vi "Generate Simulated Data v2.0.vi"(0 "Sample_Rate":dbl, 1 "A_1X":dbl, 5 "Total_Samples in":i64, 7 "Samples":i32, 9 "f_1X":dbl, 11 "error in (no error)":errorcluster, 12 "A_2X":dbl) -> (4 "Y":dbl[](array[numeric]), 6 "Total_Samples out":i64, 15 "error out":errorcluster)   [LabVIEW 2026, in "Acquisition.lvlib"]
uses:
  Acquisition.lvlib
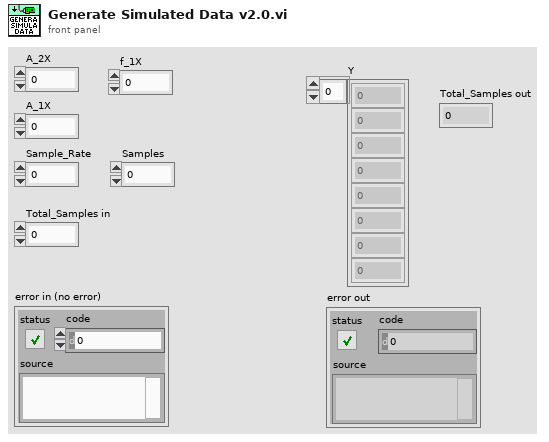
[diagram p1: front panel]
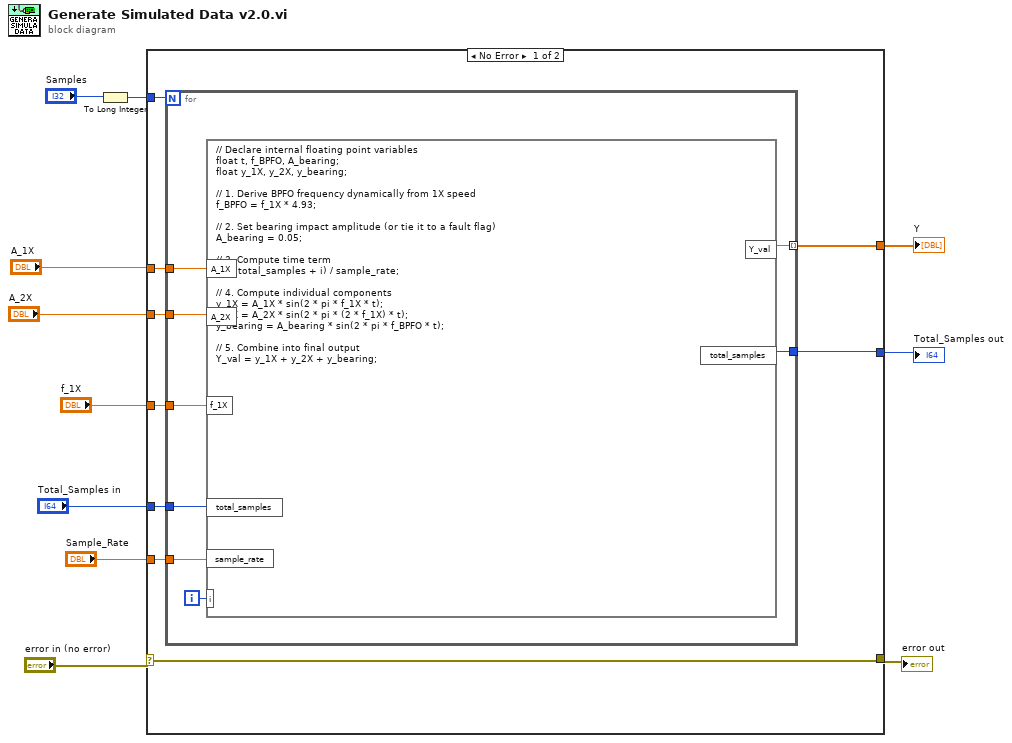
[diagram p0: block diagram]
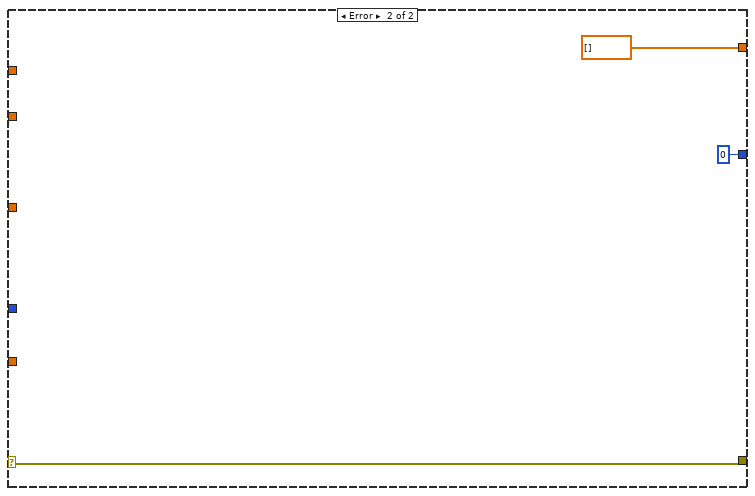
[diagram p2: hidden frame]
diagram:
  n1 = To Long Integer(number="Samples") -> (32bit integer=w3:i32)
  n2 = case shown="No Error" "error in (no error)" {
    selector: "error in (no error)" -> [w16 w31]
    tunnel: "Sample_Rate" -> [w20 _]
    tunnel: "Total_Samples in" -> [w19 _]
    tunnel: "A_1X" -> [w18 _]
    tunnel: "f_1X" -> [w17 _]
    tunnel: [w16 w31] -> w6
    tunnel: [w15 dbl[] []] -> w5
    tunnel: w3 -> [w14 _]
    tunnel: [w13 i64 0] -> w2
    tunnel: "A_2X" -> [w12 _]
    frame No Error {
      n3 = for {
        N: w14 -> [_]
        tunnel: w20 -> [w28]
        tunnel: w19 -> [w27]
        tunnel: w18 -> [w26]
        tunnel: w17 -> [w25]
        tunnel: [w24] -> w15 mode=indexing
        tunnel: [w22] -> w13
        tunnel: w12 -> [w21]
        i -> [w23]
        n4 = formula code="// Declare internal floating point variables\nfloat t, f_BPFO, A_bearing;\nfloat y_1X, y_2X, y_bearing;\n\n// 1. Derive BPFO frequency dynamically from 1X speed\nf_BPFO = f_1X * 4.93; \n\n// 2. Set bearing impact amplitude (or tie it to a fault flag)\nA_bearing = 0.05; \n\n// 3. Compute time term\nt = (total_samples + i) / sample_rate;\n\n// 4. Compute individual components\ny_1X = A_1X * sin(2 * pi * f_1X * t);\ny_2X = A_2X * sin(2 * pi * (2 * f_1X) * t);\ny_bearing = A_bearing * sin(2 * pi * f_BPFO * t);\n\n// 5. Combine into final output\nY_val = y_1X + y_2X + y_bearing;"("f_1X"=w25, "A_1X"=w26, "sample_rate"=w28, "total_samples"=w27, "i"=w23, "A_2X"=w21) -> ("Y_val"=w24:dbl, "total_samples"=w22:i64)
      }
    }
    frame Error {
    }
  }
  "error out" <- w6
  "Y" <- w5
  "Total_Samples out" <- w2
